vi "Engine-ChannelNames.vi"(11 "DSI Reference":refnum<class "DCM-DSI.lvclass">) -> ()   [LabVIEW 2016, in "DSI-RT.lvlib"]
uses:
  DSI-RT.lvlib
  Classes/DCM-DSI/DCM-DSI.lvclass
  <vilib>/Powertrain Controls/Device Drivers/DCM/Rev0/RT/DCM - RT.lvclass/DCM - RT.ctl
  <vilib>/Powertrain Controls/Device Drivers/DCM/Rev0/RT/Read Stop Target.vi
  Classes/DCM-DSI/Read DCM Ref.vi
  Classes/DCM-DSI/Read Channels.vi
  <vilib>/Powertrain Controls/Device Drivers/DCM/Rev0/RT/DCM - RT.lvclass
  <vilib>/addons/Software Calibration Management/xSCM/CalPoint.xnode
  <vilib>/addons/Software Calibration Management/xSCM/ni_scm.dll
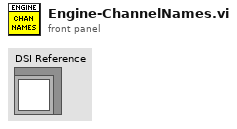
[diagram p1: front panel]
types:
  T1 = typedef "DCM-DSI.lvclass/Channel.ctl" = cluster{"Name":string, "Unit":string, "Value":sgl}
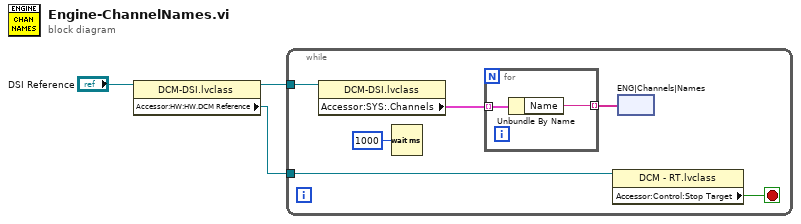
[diagram p0: block diagram]
diagram:
  n1 = property class="DCM-DSI.lvclass"(reference="DSI Reference") -> (reference out=w2:refnum<class "DCM-DSI.lvclass">, "Accessor:HW:HW.DCM Reference"=w1:refnum<class "DCM - RT.lvclass">)  [unwired: 1 in, 1 out]
  n2 = while {
    tunnel: w2 -> [w6]
    tunnel: w1 -> [w5]
    stop <- w4 stop-if-true
    n3 = property class="DCM-DSI.lvclass"(reference=w6) -> ("Accessor:SYS:.Channels"=w7:T1[])  [unwired: 1 in, 2 out]
    n4 = Wait (ms)(milliseconds to wait=u32 1000) -> ()  [unwired: 1 out]
    n5 = for {
      tunnel: w7 -> [w16] mode=indexing
      tunnel: [w15] -> w8 mode=indexing
      n6 = Unbundle By Name(w16) -> ("Name"=w15:string)
    }
    n7 = property class="DCM - RT.lvclass"(reference=w5) -> ("Accessor:Control:Stop Target"=w4:bool)  [unwired: 1 in, 2 out]
    n8 = xnode "ENG|Channels|Names"("Value"=w8) -> ()
  }
